vi "探头校准标准值设置.vi"(7 "校准参数":u16(ring) caption="校准参数：" items=["pH", "DO", "浊度", "电导率", "叶绿素a", "藻密度", "ORP", "DO2", "氯化物"], 9 "标液三":sgl, 10 "标液二":sgl, 11 "标液一":sgl) -> ()   [LabVIEW 2016, in "斯坦道多参数.lvlib"]
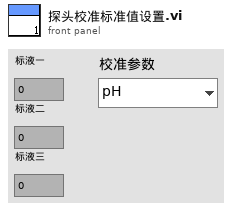
[diagram p1: front panel]
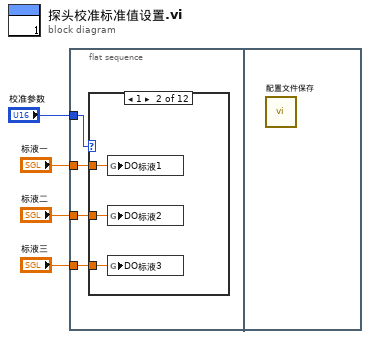
[diagram p0: block diagram]
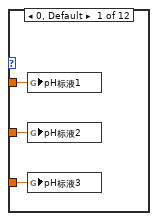
[diagram p2: hidden frame]
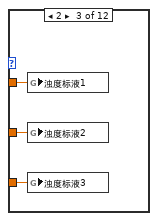
[diagram p3: hidden frame]
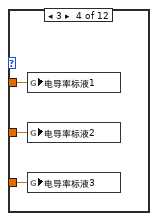
[diagram p4: hidden frame]
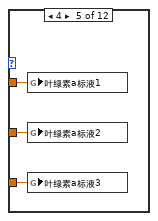
[diagram p5: hidden frame]
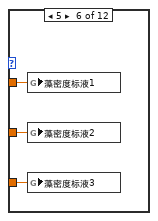
[diagram p6: hidden frame]
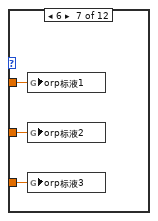
[diagram p7: hidden frame]
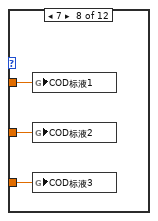
[diagram p8: hidden frame]
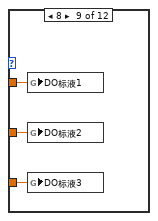
[diagram p9: hidden frame]
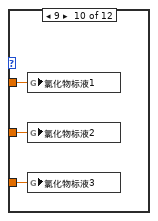
[diagram p10: hidden frame]
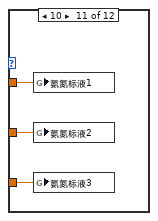
[diagram p11: hidden frame]
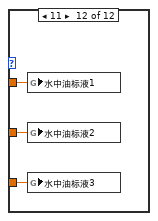
[diagram p12: hidden frame]
diagram:
  n1 = flat-sequence {
    tunnel: "校准参数" -> [w8]
    tunnel: "标液一" -> [w7]
    tunnel: "标液二" -> [w6]
    tunnel: "标液三" -> [w5]
    frame #0 {
      n2 = case shown="1" w8 {
        tunnel: w7 -> [w11 w14 w17 w20 w23 w26 w29 w32 w35 w38 w41 w44]
        tunnel: w6 -> [w10 w13 w16 w19 w22 w25 w28 w31 w34 w37 w40 w43]
        tunnel: w5 -> [w9 w12 w15 w18 w21 w24 w27 w30 w33 w36 w39 w42]
        frame 0, Default {
          n3 = global write "断电保存变量.vi" "pH标液1"(w11) -> ()
          n4 = global write "断电保存变量.vi" "pH标液2"(w10) -> ()
          n5 = global write "断电保存变量.vi" "pH标液3"(w9) -> ()
        }
        frame 1 {
          n6 = global write "断电保存变量.vi" "DO标液1"(w14) -> ()
          n7 = global write "断电保存变量.vi" "DO标液2"(w13) -> ()
          n8 = global write "断电保存变量.vi" "DO标液3"(w12) -> ()
        }
        frame 2 {
          n9 = global write "断电保存变量.vi" "浊度标液1"(w17) -> ()
          n10 = global write "断电保存变量.vi" "浊度标液2"(w16) -> ()
          n11 = global write "断电保存变量.vi" "浊度标液3"(w15) -> ()
        }
        frame 3 {
          n12 = global write "断电保存变量.vi" "电导率标液1"(w20) -> ()
          n13 = global write "断电保存变量.vi" "电导率标液2"(w19) -> ()
          n14 = global write "断电保存变量.vi" "电导率标液3"(w18) -> ()
        }
        frame 4 {
          n15 = global write "断电保存变量.vi" "叶绿素a标液1"(w23) -> ()
          n16 = global write "断电保存变量.vi" "叶绿素a标液2"(w22) -> ()
          n17 = global write "断电保存变量.vi" "叶绿素a标液3"(w21) -> ()
        }
        frame 5 {
          n18 = global write "断电保存变量.vi" "藻密度标液1"(w26) -> ()
          n19 = global write "断电保存变量.vi" "藻密度标液2"(w25) -> ()
          n20 = global write "断电保存变量.vi" "藻密度标液3"(w24) -> ()
        }
        frame 6 {
          n21 = global write "断电保存变量.vi" "orp标液1"(w29) -> ()
          n22 = global write "断电保存变量.vi" "orp标液2"(w28) -> ()
          n23 = global write "断电保存变量.vi" "orp标液3"(w27) -> ()
        }
        frame 7 {
          n24 = global write "断电保存变量.vi" "COD标液1"(w32) -> ()
          n25 = global write "断电保存变量.vi" "COD标液2"(w31) -> ()
          n26 = global write "断电保存变量.vi" "COD标液3"(w30) -> ()
        }
        frame 8 {
          n27 = global write "断电保存变量.vi" "DO标液1"(w35) -> ()
          n28 = global write "断电保存变量.vi" "DO标液2"(w34) -> ()
          n29 = global write "断电保存变量.vi" "DO标液3"(w33) -> ()
        }
        frame 9 {
          n30 = global write "断电保存变量.vi" "氯化物标液1"(w38) -> ()
          n31 = global write "断电保存变量.vi" "氯化物标液2"(w37) -> ()
          n32 = global write "断电保存变量.vi" "氯化物标液3"(w36) -> ()
        }
        frame 10 {
          n33 = global write "断电保存变量.vi" "氨氮标液1"(w41) -> ()
          n34 = global write "断电保存变量.vi" "氨氮标液2"(w40) -> ()
          n35 = global write "断电保存变量.vi" "氨氮标液3"(w39) -> ()
        }
        frame 11 {
          n36 = global write "断电保存变量.vi" "水中油标液1"(w44) -> ()
          n37 = global write "断电保存变量.vi" "水中油标液2"(w43) -> ()
          n38 = global write "断电保存变量.vi" "水中油标液3"(w42) -> ()
        }
      }
    }
    frame #1 {
      n39 = call "配置文件保存.vi"() -> ()  [unwired: 12 in]
    }
  }
